vi "Profile_generator_core.vi"(11 "Motion profile inputs":T2={"Max Acceleration (inches/sec^2)"=0.0, "Maximun Speed (IPS)"=0.0, "Control loop Hz"=100.0, "Distance in inches"=0.0, "Max \"Jerk\" (inches/sec^3)"=0.0}) -> (3 "Motion profile outputs":T1)   [LabVIEW 2017, in "labview-standard-library.lvlib"]
uses:
  labview-standard-library.lvlib
  Motion_Profile_Inputs.ctl
  Motion_Profile_Outputs.ctl
panel:
  out "Speed Graph 2":dbl[](graph)
  out "Acceleration Graph":dbl[](graph)
  out "Speed Graph":dbl[](graph)
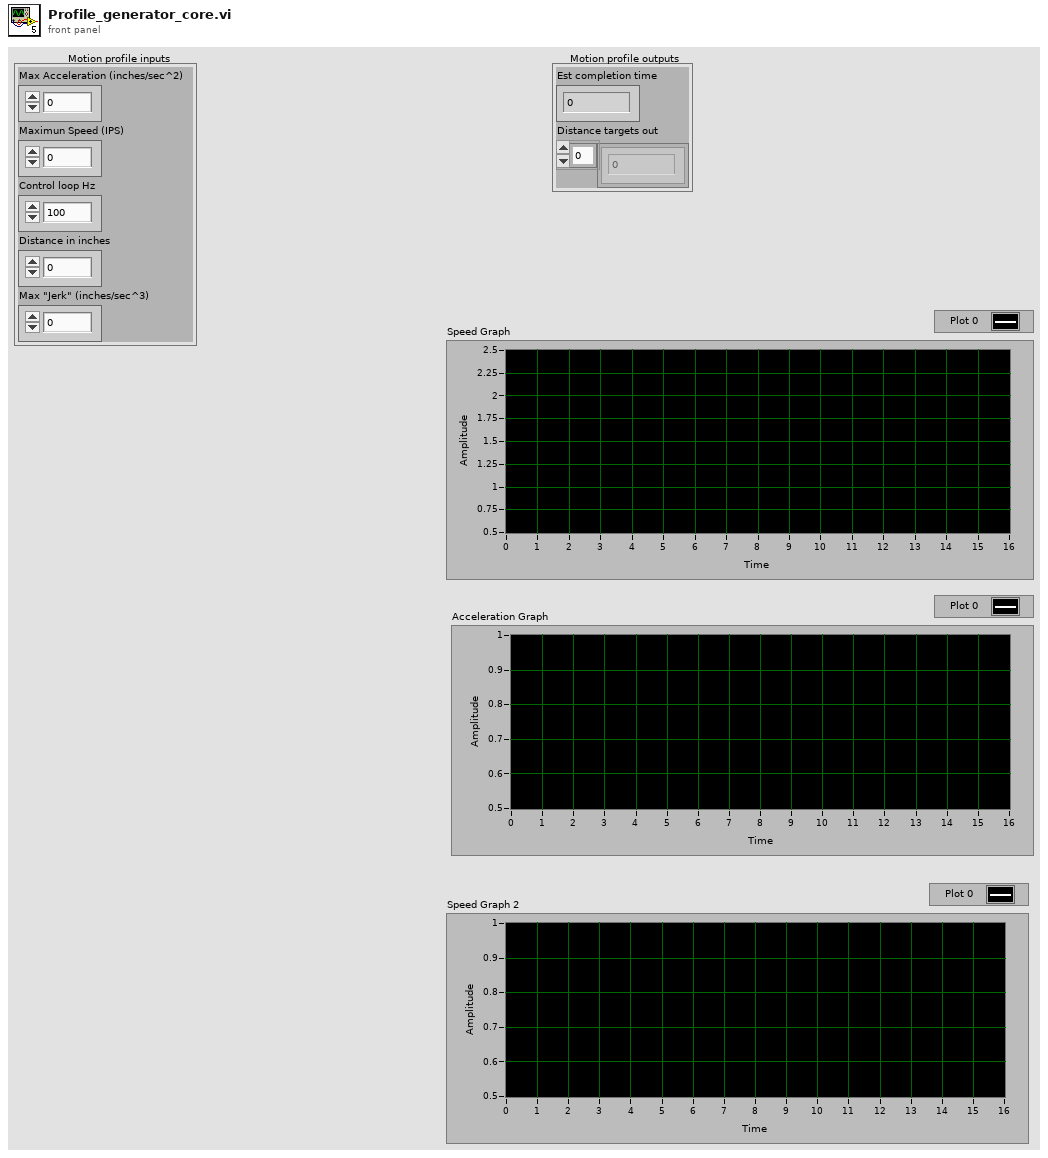
[diagram p1: front panel]
types:
  T1 = typedef "labview-standard-library.lvlib/Motion_Profile_Outputs.ctl" = cluster{"Est completion time":dbl, "Distance targets out":dbl[]}
  T2 = typedef "labview-standard-library.lvlib/Motion_Profile_Inputs.ctl" = cluster{"Max Acceleration (inches/sec^2)":dbl, "Maximun Speed (IPS)":dbl, "Control loop Hz":dbl, "Distance in inches":dbl, "Max \"Jerk\" (inches/sec^3)":dbl}
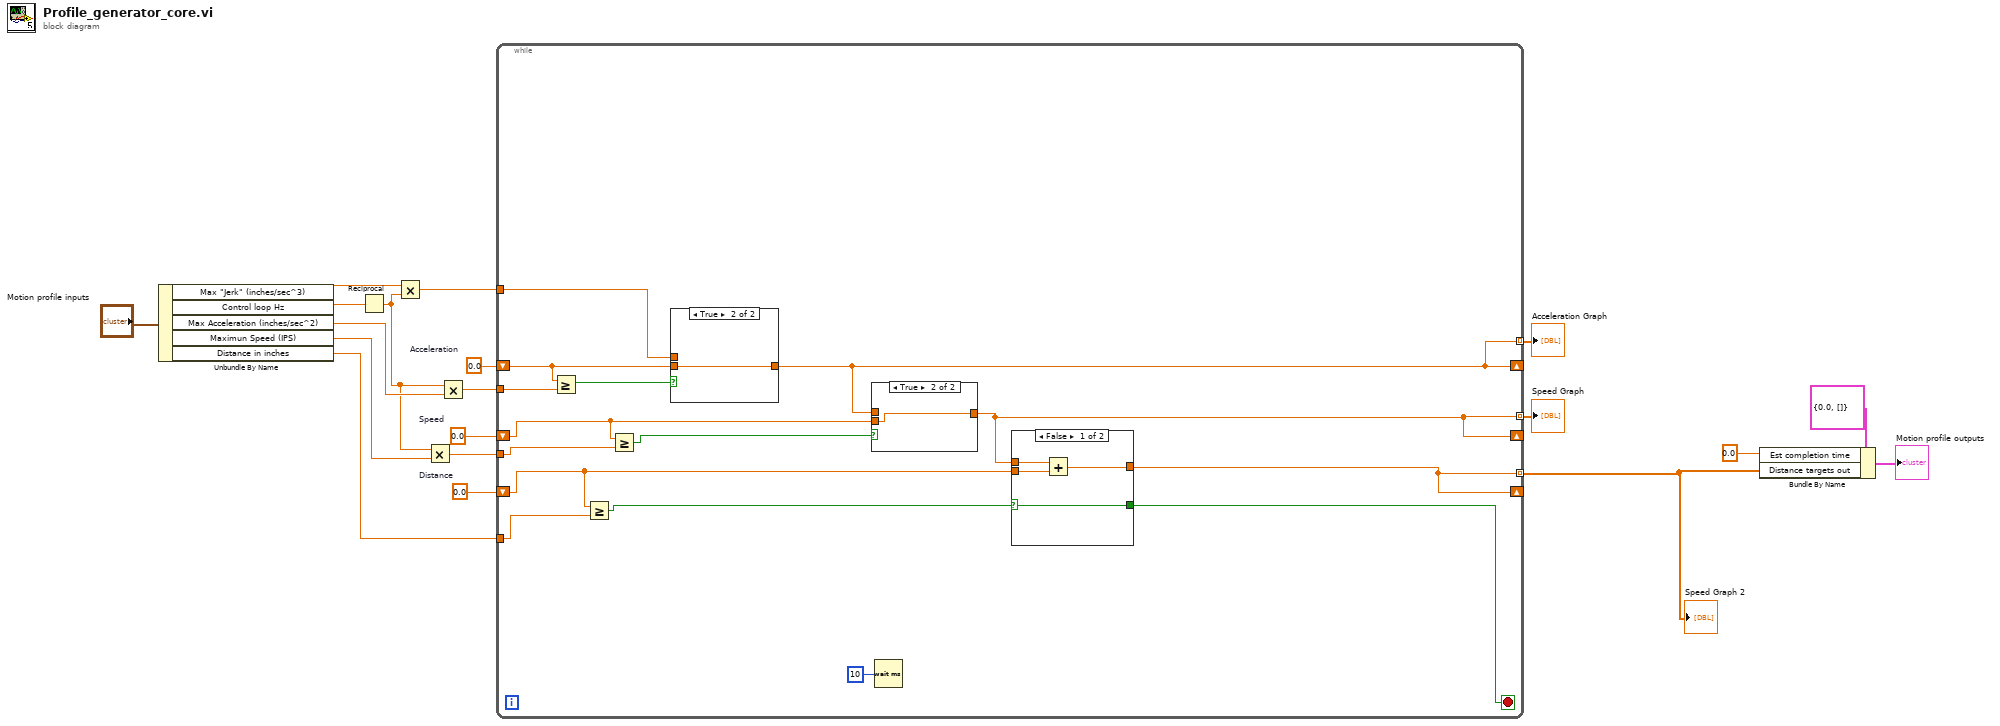
[diagram p0: block diagram]
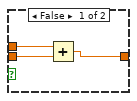
[diagram p2: hidden frame]
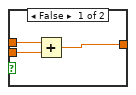
[diagram p3: hidden frame]
diagram:
  w5 = 0.0  # Speed
  w12 = 0.0  # Distance
  w15 = 0.0  # Acceleration
  n1 = Unbundle By Name("Motion profile inputs") -> ("Max \"Jerk\" (inches/sec^3)"=w14:dbl, "Control loop Hz"=w16:dbl, "Max Acceleration (inches/sec^2)"=w10:dbl, "Maximun Speed (IPS)"=w7:dbl, "Distance in inches"=w11:dbl)
  n2 = Reciprocal(x=w16) -> (1/x=w6:dbl)
  n3 = Multiply(x=w14, y=w6) -> (x*y=w13:dbl)
  n4 = Multiply(x=w6, y=w7) -> (x*y=w8:dbl)
  n5 = Multiply(x=w6, y=w10) -> (x*y=w9:dbl)
  n6 = while {
    shift-right: [w31] -> _
    shift-left: w15 -> [w21]
    tunnel: w13 -> [w33]
    shift-right: [w32] -> _
    shift-left: w12 -> [w30]
    tunnel: w11 -> [w29]
    tunnel: w9 -> [w22]
    tunnel: w8 -> [w24]
    shift-right: [w26] -> _
    shift-left: w5 -> [w25]
    tunnel: [w32] -> w1 mode=indexing
    tunnel: [w26] -> w3 mode=indexing
    tunnel: [w31] -> w2 mode=indexing
    stop <- w27 stop-if-true
    n7 = Greater Or Equal?(x=w21, y=w22) -> (x >= y?=w20:bool)
    n8 = Greater Or Equal?(x=w30, y=w29) -> (x >= y?=w28:bool)
    n9 = Greater Or Equal?(x=w25, y=w24) -> (x >= y?=w23:bool)
    n10 = case shown="True" w20 {
      tunnel: w33 -> [w37 _]
      tunnel: [w36 w38] -> w31
      tunnel: w21 -> [w35 w38]
      frame False {
        n11 = Add(x=w37, y=w35) -> (x+y=w36:dbl)
      }
      frame True {
      }
    }
    n12 = case shown="True" w23 {
      tunnel: w25 -> [w41 w42]
      tunnel: [w40 w42] -> w26
      tunnel: w31 -> [w39 _]
      frame False {
        n13 = Add(x=w39, y=w41) -> (x+y=w40:dbl)
      }
      frame True {
      }
    }
    n14 = Wait (ms)(milliseconds to wait=u32 10) -> ()  [unwired: 1 out]
    n15 = case shown="False" w28 {
      selector: w28 -> [w43 w47]
      tunnel: w30 -> [w46 w48]
      tunnel: [w45 w48] -> w32
      tunnel: w26 -> [w44 _]
      tunnel: [w43 w47] -> w27
      frame False {
        n16 = Add(x=w44, y=w46) -> (x+y=w45:dbl)
      }
      frame True {
      }
    }
  }
  "Speed Graph" <- w3
  "Acceleration Graph" <- w2
  "Speed Graph 2" <- w1
  n17 = Bundle By Name(cluster=T1 {"Est completion time"=0.0, "Distance targets out"=[]} ("Motion profile outputs 2"), "Est completion time"=0.0, "Distance targets out"=w1) -> (→"Motion profile outputs":T1)
